vi "optimization2_thirdround.vi"() -> ()   [LabVIEW 2020]
uses:
  <vilib>/gmath/GlobalOptimization.llb/DE_Stopping Criteria.ctl
  <vilib>/gmath/GlobalOptimization.llb/DE_Settings.ctl
  <vilib>/gmath/GlobalOptimization.llb/DE_Bound Mapping Method.ctl
  <vilib>/gmath/GlobalOptimization.llb/DE_Mutation Method.ctl
  <vilib>/gmath/GlobalOptimization.llb/DE_Crossover Method.ctl
  <vilib>/gmath/NI_AAL_GlobalOptimization.lvlib
panel:
  in  "Bounds":cluster{"Min":dbl[], "Max":dbl[]}={"Min"=[0.475, 0.55, -0.03, -0.008, 1125.3, 0.1824, 4.543, 1125.7], "Max"=[0.48, 0.56, -0.028, -0.007, 1125.5, 0.18259, 4.544, 1125.8]}
  in  "Image acquisition time (ms)":dbl=76.0
  in  "Flyback time (ms)":dbl=24.0
  out "Minimum":dbl[](array[numeric])=[0.46683235098170606, 0.5199856500261317, -0.02901472423242877, -0.014679196332125671, -0.291480008210523, 116.68539163396477, -108.39593902792714, 0.643464388078615]
  out "F(Minimum)":dbl[](array[numeric])=[5.619076172673733]
  in  "DE settings":T1={"population size"=10, "scale factor"=0.9, "crossover probability"=0.95, "bound mapping method"=1, "mutation method"=0, "crossover method"=0} {"crossover method" items=["Uniform", "Exponential"]; "mutation method" items=["Random", "Either Or", "Best", "Target to Best"]; "bound mapping method" items=["None", "Random between Bounds and Values", "Re-Initialize"]}
  in  "stopping criteria":T5={"max iterations"=10, "max function calls"=-1, "max time (sec)"=-1.0}
  out "number of function calls":i32=110
  out "VI Type":T6(ring)=enum."Standard VI"
  # "lambda x: 1125.401403483864 * np.sin(0.18254813799004393 * x + 4.543945659094395) + 1125.7766598429089])"
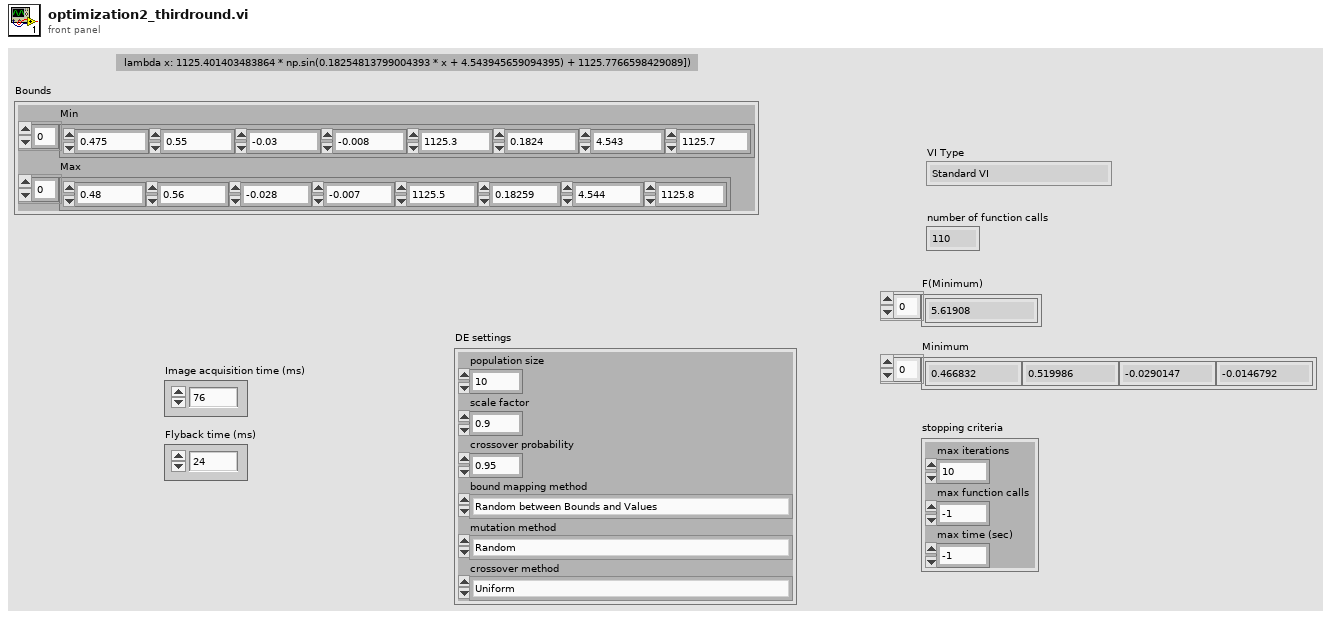
[diagram p1: front panel]
types:
  T1 = typedef "NI_AAL_GlobalOptimization.lvlib/DE_Settings.ctl" = cluster{"population size":i32, "scale factor":dbl, "crossover probability":dbl, "bound mapping method":T2, "mutation method":T3, "crossover method":T4}
  T2 = typedef "NI_AAL_GlobalOptimization.lvlib/DE_Bound Mapping Method.ctl" = u16
  T3 = typedef "NI_AAL_GlobalOptimization.lvlib/DE_Mutation Method.ctl" = u16
  T4 = typedef "NI_AAL_GlobalOptimization.lvlib/DE_Crossover Method.ctl" = u16
  T5 = typedef "NI_AAL_GlobalOptimization.lvlib/DE_Stopping Criteria.ctl" = cluster{"max iterations":i32, "max function calls":i32, "max time (sec)":dbl}
  T6 = enum32{"invalid VI type", "Standard VI", "Control VI", "Global VI", "Polymorphic VI", "Configuration VI", "SubSystem", "Facade VI", "Method VI", "Statechart Diagram VI"}
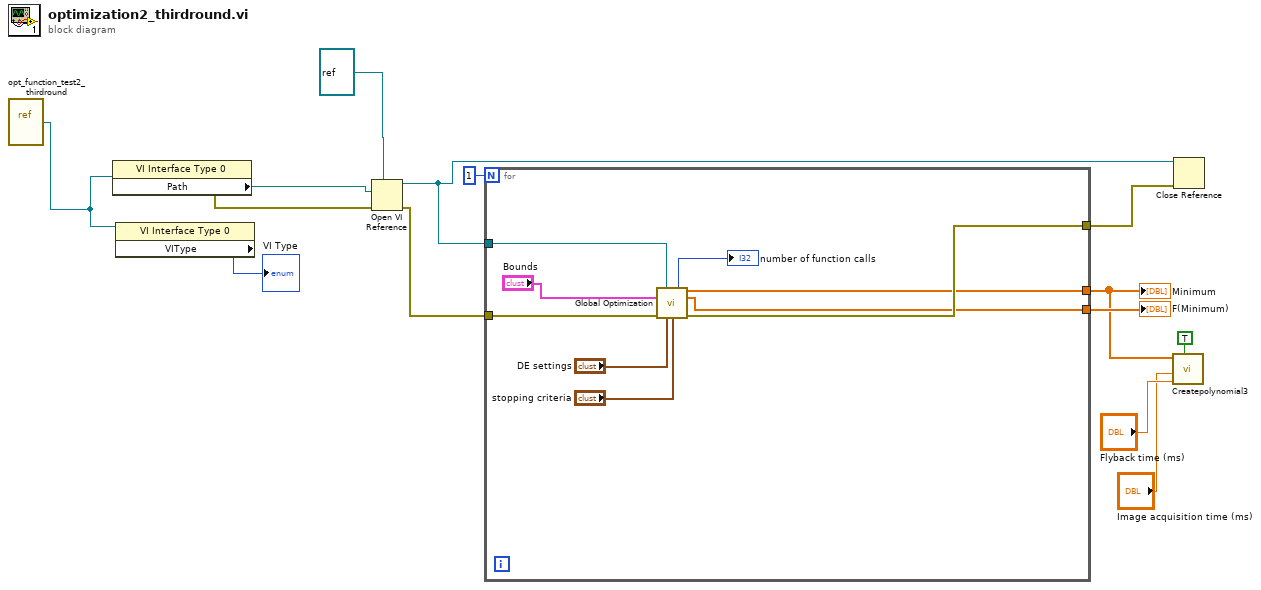
[diagram p0: block diagram]
diagram:
  n1 = vi-ref "opt_function_test2_thirdround.vi"() -> (w2:refnum<vi>)
  n2 = property class="VI Interface Type 0"(reference=w2) -> (error out=w4:errorcluster, "Path"=w5:path)  [unwired: 1 in, 1 out]
  n3 = property class="VI Interface Type 0"(reference=w2) -> ("VIType"=→"VI Type":T6)  [unwired: 1 in, 2 out]
  n4 = Open VI Reference(type specifier VI Refnum (for type only)=refnum<vi> refnum, vi path=w5, error in (no error)=w4) -> (vi reference=w3:refnum<vi>, error out=w11:errorcluster)  [unwired: 3 in]
  n5 = for {
    N: 1 -> [_]
    tunnel: [w20] -> w12
    tunnel: w11 -> [w19]
    tunnel: [w18] -> w9
    tunnel: [w17] -> w10
    tunnel: w3 -> [w16]
    n6 = call <vilib>:"Global Optimization.vi"("objective and constraint function"=w16, "Bounds"="Bounds", "error in (no error)"=w19, "DE settings"="DE settings", "stopping criteria"="stopping criteria") -> ("number of function calls"=→"number of function calls":i32, "Minimum"=w18:dbl[], "F(Minimum)"=w17:dbl[], "error out"=w20:errorcluster)  [unwired: 6 in, 1 out]
  }
  "F(Minimum)" <- w10
  "Minimum" <- w9
  n7 = call "Createpolynomial3.vi"("Save calibration"=TRUE, "Flyback (ms)"="Flyback time (ms)", "Acquisition time (ms)"="Image acquisition time (ms)", "P(x)"=w9) -> ()  [unwired: 7 in, 1 out]
  n8 = Close Reference(reference=w3, error in (no error)=w12) -> ()  [unwired: 1 out]
